vi "GLdrv_Open_TCPIP.vi"(0 "address":string, 5 "remote port":u16) -> (4 "Connection ID":T1, 15 "error out":errorcluster)   [LabVIEW 2017]
uses:
  ConnectionID.ctl
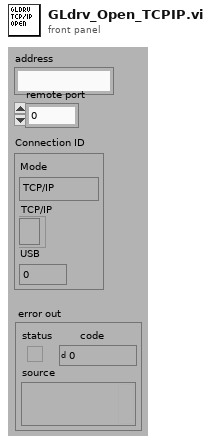
[diagram p1: front panel]
types:
  T1 = typedef "ConnectionID.ctl" = cluster{"Mode":enum16{"TCP/IP", "USB"}, "TCP/IP":refnum<k5>, "USB":i32}
  T2 = cluster{"Mode":enum16{"TCP/IP", "USB"}, "connection ID":refnum<k5>, "USB":i32}
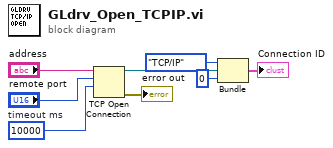
[diagram p0: block diagram]
diagram:
  w1 = 10000  # timeout ms
  n1 = TCP Open Connection(address="address", remote port or service name="remote port", timeout ms (60000)=w1) -> (connection ID=w4:refnum<k5>, error out=→"error out":errorcluster)  [unwired: 2 in]
  n2 = Bundle("Mode"=enum16{"TCP/IP", "USB"}."TCP/IP", "connection ID"=w4, "USB"=0) -> (→"Connection ID":T2)  [unwired: 1 out]
